vi "Get Bounds.vi"   [LabVIEW 2020, in "Camera.lvclass"]
uses:
  Camera.lvclass
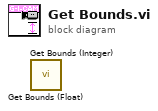
[diagram p0: block diagram]
diagram:
  n1 = call "Get Bounds (Float).vi"() -> ()  [unwired: 8 in, 4 out]
  n2 = call "Get Bounds (Integer).vi"() -> ()  [unwired: 8 in, 4 out]
